vi "Instrument Status.vi"(8 "error in (no error)":errorcluster, 11 "VISA resource name":refnum<visa-resource-name>) -> (0 "error out":errorcluster, 1 "Emulation Mode":u16(ring) items=["None (335)", "331", "332"], 2 "Lock Code":u16=123, 3 "VISA resource name out":refnum<visa-resource-name>, 4 "PID Control Scaling":u16(ring) items=["335 (Temperature)", "331/332 (Sensor)"], 5 "Keypad Locked":bool, 6 "Remote Interface Mode":u16(ring) items=["Local", "Remote", "Remote with local lockout"])   [LabVIEW 2019, in "Lake Shore 335.lvlib"]
doc: "Returns various instrument settings. Parameters returned are;\nRemote interface mode, key status, keypad lock out, and emulation information. \n\n<B>Note - If this VI is used while the 335 is in 331 or 332 emulation mode and the 335 Initialize VI is used, be sure to turn off ID Query. </B>"
uses:
  Lake Shore 335.lvlib
  Instance           1 25Saved   Instrument Status .vi
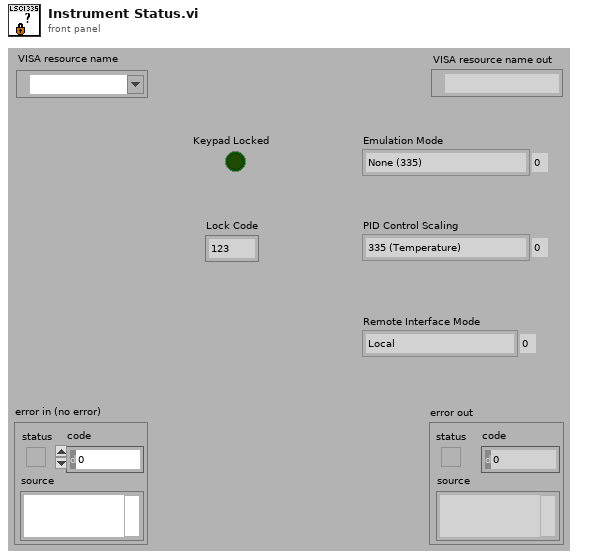
[diagram p1: front panel]
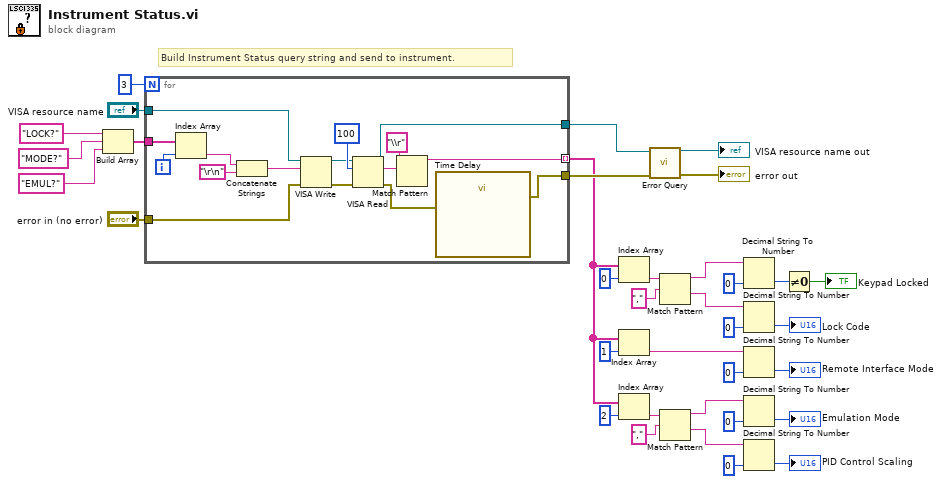
[diagram p0: block diagram]
diagram:
  # "Build Instrument Status query string and send to instrument."
  n1 = Build Array("LOCK?", "MODE?", "EMUL?") -> (w33:string[])
  n2 = for {
    N: 3 -> [_]
    tunnel: [w45] -> w12
    tunnel: [w40] -> w13
    tunnel: "VISA resource name" -> [w44]
    tunnel: "error in (no error)" -> [w43]
    tunnel: w33 -> [w42]
    tunnel: [w41] -> w9 mode=indexing
    i -> [w46]
    n3 = Index Array(array=w42, index=w46) -> (element=w36:string)
    n4 = Concatenate Strings(w36, "\r\n") -> (w37:string)
    n5 = VISA Write(VISA resource name=w44, write buffer=w37, error in (no error)=w43) -> (VISA resource name out=w48:refnum<visa-resource-name>, error out=w47:errorcluster)  [unwired: 1 out]
    n6 = VISA Read(VISA resource name=w48, byte count=100, error in (no error)=w47) -> (VISA resource name out=w45:refnum<visa-resource-name>, read buffer=w50:string, error out=w39:errorcluster)  [unwired: 1 out]
    n7 = Match Pattern(string=w50, regular expression="\\r") -> (before substring=w41:string)  [unwired: 1 in, 3 out]
    n8 = call "Time Delay"("error in (no error)"=w39) -> ("error out"=w40:errorcluster)  [unwired: 10 in]
  }
  n9 = Index Array(array=w9, index=0) -> (element=w28:string)
  n10 = Index Array(array=w9, index=1) -> (element=w25:string)
  n11 = Index Array(array=w9, index=2) -> (element=w7:string)
  n12 = call "Error Query.vi"("error in (no error)"=w13, "VISA resource name"=w12) -> ("error out"=→"error out":errorcluster, "VISA resource name out"=→"VISA resource name out":refnum<visa-resource-name>)  [unwired: 7 in, 1 out]
  n13 = Match Pattern(string=w28, regular expression=",") -> (before substring=w20:string, after substring=w19:string)  [unwired: 1 in, 2 out]
  n14 = Match Pattern(string=w7, regular expression=",") -> (before substring=w4:string, after substring=w3:string)  [unwired: 1 in, 2 out]
  n15 = Decimal String To Number(string=w20, default (0L)=u16 0) -> (number=w21:u16)  [unwired: 1 in, 1 out]
  n16 = Decimal String To Number(string=w19, default (0L)=u16 0) -> (number=→"Lock Code":u16)  [unwired: 1 in, 1 out]
  n17 = Decimal String To Number(string=w25, default (0L)=u16 0) -> (number=→"Remote Interface Mode":u16)  [unwired: 1 in, 1 out]
  n18 = Decimal String To Number(string=w4, default (0L)=u16 0) -> (number=→"Emulation Mode":u16)  [unwired: 1 in, 1 out]
  n19 = Decimal String To Number(string=w3, default (0L)=u16 0) -> (number=→"PID Control Scaling":u16)  [unwired: 1 in, 1 out]
  n20 = Not Equal To 0?(x=w21) -> (x != 0?=→"Keypad Locked":bool)
